vi "Quit.vi"(8 "No Error":errorcluster) -> (0 "error out":errorcluster)   [LabVIEW 2024, in "SDL3.lvlib" / "Init.lvlib"]
doc: "Clean up all initialized subsystems."
uses:
  Init.lvlib
  _LV-SDL3/Lib/SDL3-32.dll
panel:
  # "https://wiki.libsdl.org/SDL3/SDL_Quit"
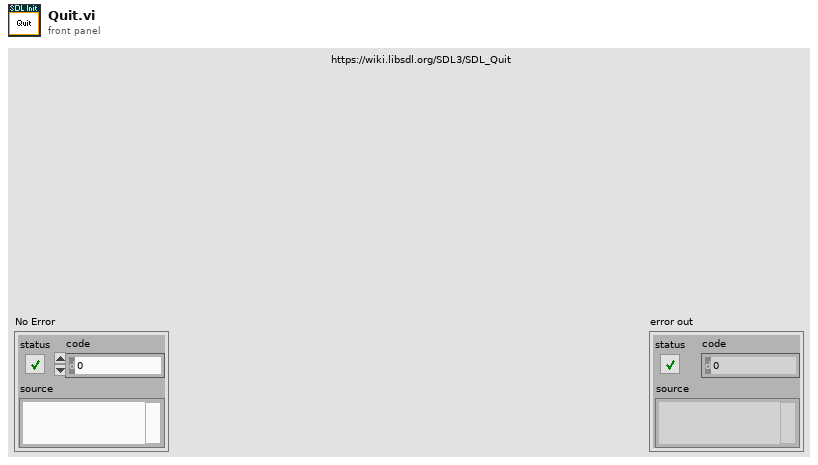
[diagram p1: front panel]
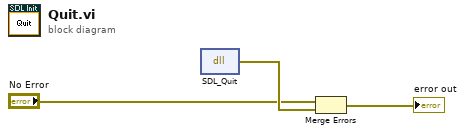
[diagram p0: block diagram]
diagram:
  n1 = dll-call lib="C:/Users/Thomas/Documents/Projects/_LV-SDL3/Lib/SDL3-*.*" fn="SDL_Quit"() -> (error out=w3:errorcluster)  [unwired: 4 in, 1 out]
  n2 = Merge Errors("No Error", w3) -> (→"error out":errorcluster)
